vi "Lab04 JohnDoldol.vi"() -> ()   [LabVIEW 2016]
uses:
  <vilib>/DAQmx/read.llb/DAQmx Read (Analog DBL 1Chan 1Samp).vi
  <vilib>/DAQmx/miscellaneous.llb/DAQmx Fill In Error Info.vi
panel:
  in  "stop 2":bool
  out "Thermometer":dbl(slide) scale=0.0..100.0
  out "Waveform Chart":dbl(graph)
  out "data":dbl format="%0.2f"
  in  "task/channels in":refnum<k21>
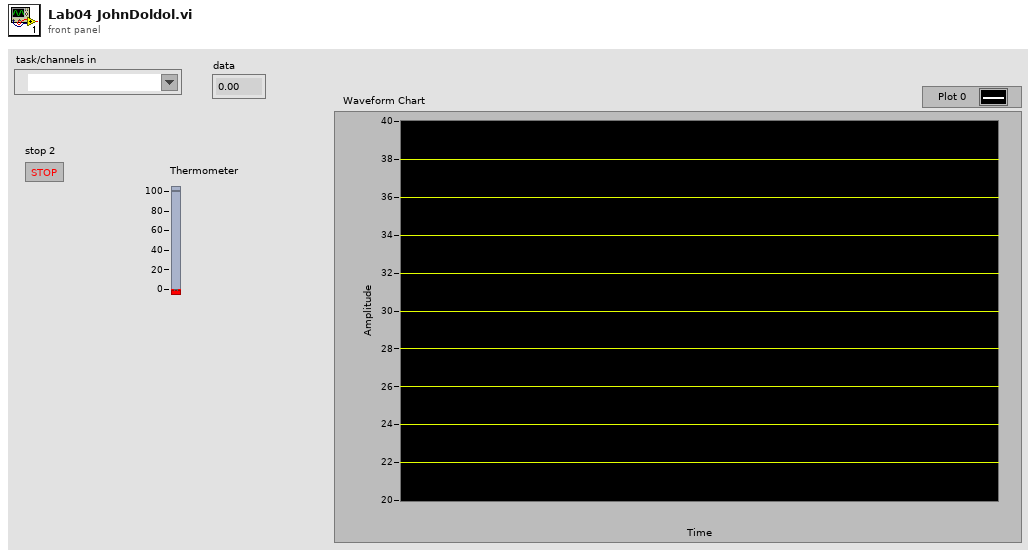
[diagram p1: front panel]
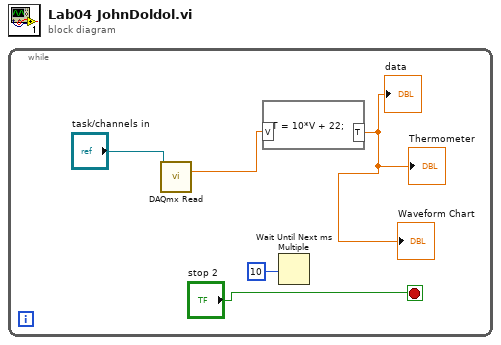
[diagram p0: block diagram]
diagram:
  n1 = while {
    stop <- "stop 2" stop-if-true
    n2 = call-poly <vilib>:"DAQmx Read.vi"("task/channels in"="task/channels in") -> ("data"=w3:dbl)  [unwired: 12 in, 2 out]
    n3 = formula code="T = 10*V + 22;"("V"=w3) -> ("T"=→"data" →"Waveform Chart" →"Thermometer":dbl)
    n4 = Wait Until Next ms Multiple(millisecond multiple=10) -> ()  [unwired: 1 out]
  }
